vi "Motion Cases.vi"(6 "Motion Indicator Refnum":refnum<vi>, 8 "error in (no error)":errorcluster, 9 "Data":variant, 10 "State":T2, 11 "Hardware Settings in":refnum<class "Process Settings.lvclass">) -> (0 "error out":errorcluster, 1 "Limits":T3, 2 "Expansion Queue Element":T1, 3 "Hardware Settings out":refnum<class "Process Settings.lvclass">)   [LabVIEW 2017, in "Expansion.lvclass"]
uses:
  Expansion.lvclass
  Type Defs/Expansion State.ctl
  Process Settings/Process Settings.lvclass
  Type Defs/Limit Switches.ctl
  Type Defs/Expansion Queue Element.ctl
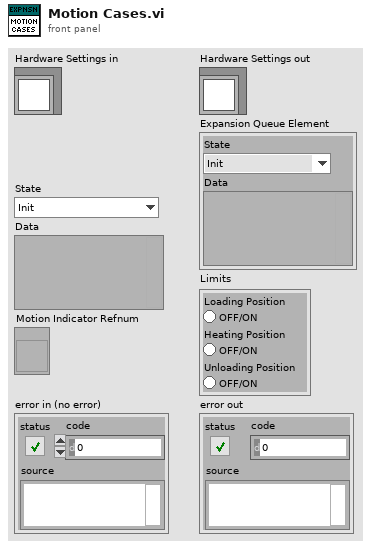
[diagram p1: front panel]
types:
  T1 = typedef "Expansion.lvclass/Expansion Queue Element.ctl" = cluster{"State":T2, "Data":variant}
  T2 = typedef "Expansion.lvclass/Expansion State.ctl" = enum16{"Init", "Update", "Go", "Move from Load to Heating", "Stop Motor", "Operate Cylinders", "Wait and Monitor", "Move from Heating to Unload", "Unload", "Move from Unload to Heating", "Move from Heating to Load", "Complete Process", "Stop", "Idle", "Error", "Shutdown"}
  T3 = typedef "Expansion.lvclass/Limit Switches.ctl" = cluster{"Loading Position":bool, "Heating Position":bool, "Unloading Position":bool}
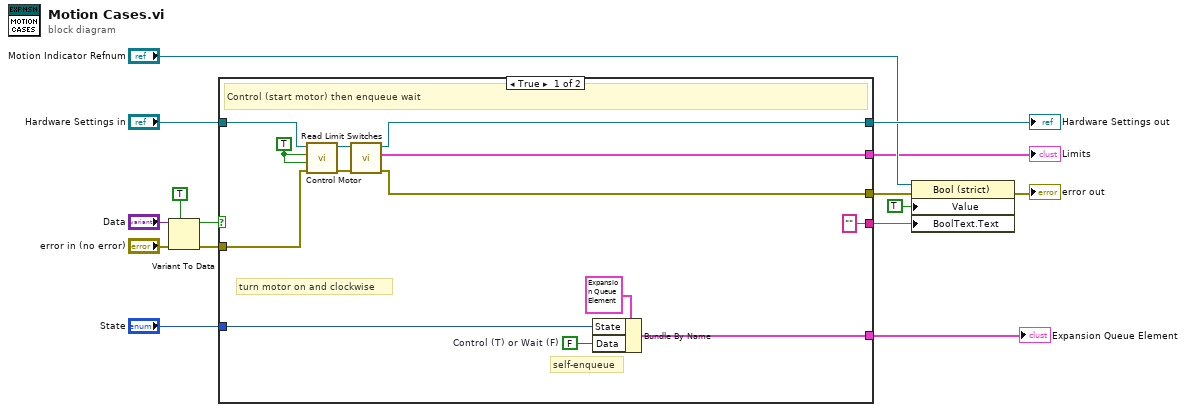
[diagram p0: block diagram]
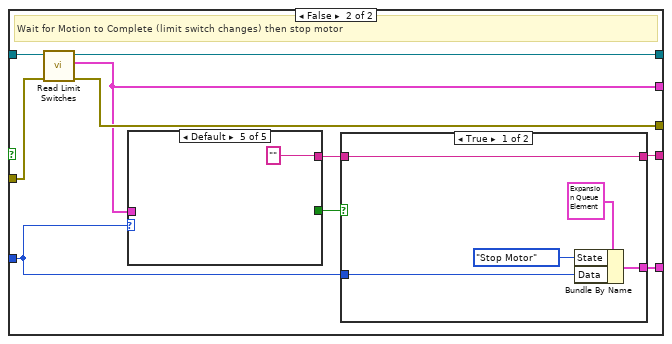
[diagram p2: hidden frame]
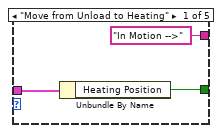
[diagram p3: hidden frame]
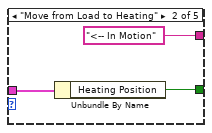
[diagram p4: hidden frame]
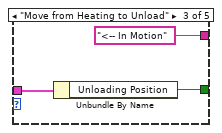
[diagram p5: hidden frame]
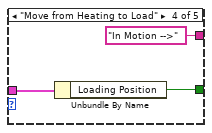
[diagram p6: hidden frame]
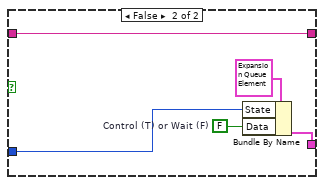
[diagram p7: hidden frame]
diagram:
  n1 = Variant To Data(error in="error in (no error)", type=TRUE, Variant="Data") -> (data=w14:bool, error out=w13:errorcluster)
  n2 = case shown="True" w14 {
    tunnel: "Hardware Settings in" -> [w28 w38]
    tunnel: [w26 w37] -> w9
    tunnel: w13 -> [w24 w36]
    tunnel: "State" -> [w21 w33]
    tunnel: [w20 w32] -> w5
    tunnel: [w19 w35] -> w6
    tunnel: [w18 w34] -> w4
    tunnel: ["" ("f") w30] -> w2
    frame True {
      w22 = FALSE  # Control (T) or Wait (F)
      w16 = TRUE
      # "self-enqueue"
      # "turn motor on and clockwise"
      # "Control (start motor) then enqueue wait"
      n3 = call "Control Motor.vi"("error in (no error)"=w24, "Motor Power"=w16, "Motor Direction"=w16, "Process Settings in"=w28) -> ("error out"=w25:errorcluster, "Process Settings out"=w27:refnum<class "Process Settings.lvclass">)  [unwired: 6 in]
      n4 = call "Read Limit Switches.vi"("error in (no error)"=w25, "Process Settings in"=w27) -> ("error out"=w18:errorcluster, "Limits"=w20:T3, "Process Settings out"=w26:refnum<class "Process Settings.lvclass">)  [unwired: 7 in]
      n5 = Bundle By Name(cluster=T1 {"State"=enum."Move from Load to Heating", "Data"=variant} ("Expansion Queue Element"), "State"=w21, "Data"=w22) -> (w19:T1)
    }
    frame False {
      # "Wait for Motion to Complete (limit switch changes) then stop motor"
      n6 = call "Read Limit Switches.vi"("error in (no error)"=w36, "Process Settings in"=w38) -> ("error out"=w34:errorcluster, "Limits"=w32:T3, "Process Settings out"=w37:refnum<class "Process Settings.lvclass">)  [unwired: 7 in]
      n7 = case shown="Default" w33 {
        tunnel: w32 -> [w41 w44 w47 w50 _]
        tunnel: [w40 w43 w46 w49 _] -> w31
        tunnel: ["In Motion -->" ("Boolean Text.Text") "<-- In Motion" ("Boolean Text.Text") "<-- In Motion" ("Boolean Text.Text") "In Motion -->" ("Boolean Text.Text") "" ("f")] -> w29
        frame "Move from Unload to Heating" {
          n8 = Unbundle By Name(w41) -> ("Heating Position"=w40:bool)
        }
        frame "Move from Load to Heating" {
          n9 = Unbundle By Name(w44) -> ("Heating Position"=w43:bool)
        }
        frame "Move from Heating to Unload" {
          n10 = Unbundle By Name(w47) -> ("Unloading Position"=w46:bool)
        }
        frame "Move from Heating to Load" {
          n11 = Unbundle By Name(w50) -> ("Loading Position"=w49:bool)
        }
        frame Default {
        }
      }
      n12 = case shown="True" w31 {
        tunnel: [w56 w61] -> w35
        tunnel: w33 -> [w53 w58]
        tunnel: [w52 w57] -> w30
        tunnel: w29 -> [w52 w57]
        frame True {
          n13 = Bundle By Name(cluster=T1 {"State"=enum."Move from Load to Heating", "Data"=variant} ("Expansion Queue Element"), "State"=Expansion_State."Stop Motor", "Data"=w53) -> (w56:T1)
        }
        frame False {
          w59 = FALSE  # Control (T) or Wait (F)
          n14 = Bundle By Name(cluster=T1 {"State"=enum."Move from Load to Heating", "Data"=variant} ("Expansion Queue Element"), "State"=w58, "Data"=w59) -> (w61:T1)
        }
      }
    }
  }
  "Hardware Settings out" <- w9
  "Expansion Queue Element" <- w6
  "Limits" <- w5
  n15 = property on="Property Node" class="Bool (strict)"(reference="Motion Indicator Refnum", error in=w4, "Value"=TRUE, "BoolText.Text"=w2) -> (error out=→"error out":errorcluster)  [unwired: 1 out]
